vi "Read Logger.vi"(8 "error in (no error)":errorcluster, 11 "Log Message in":refnum<class "Log Message.lvclass">) -> (0 "error out":errorcluster, 2 "Logger":T1, 3 "Log Message out":refnum<class "Log Message.lvclass">)   [LabVIEW 2020, in "AIM MIL-STD-1553 Engine.lvlib" / "Implementation.lvlib" / "Word Logging.lvlib" / "Log Message.lvclass"]
uses:
  Log Message.lvclass
  Logger Data Reference.ctl
  Logger Interface/Logger Interface.lvclass
  Log Message.lvclass/Log Message.ctl
  Word Logging.lvlib
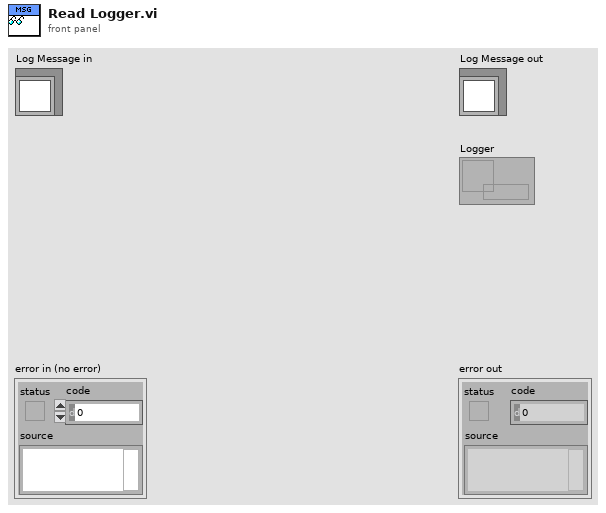
[diagram p1: front panel]
types:
  T1 = typedef "AIM MIL-STD-1553 Engine.lvlib/Implementation.lvlib/Word Logging.lvlib/Logger Data Reference.ctl" = refnum<data-value>
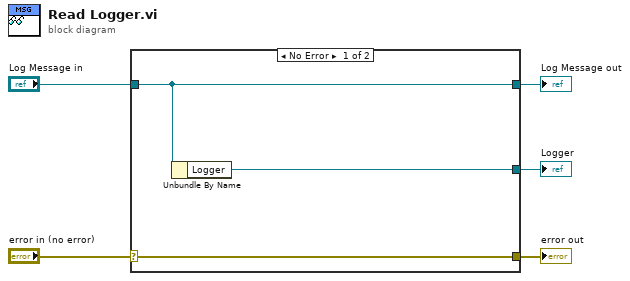
[diagram p0: block diagram]
diagram:
  n1 = case shown="No Error" "error in (no error)" {
    selector: "error in (no error)" -> [w8 w9]
    tunnel: [w8 w9] -> w4
    tunnel: [w7 w10] -> w2
    tunnel: "Log Message in" -> [w7 w10]
    tunnel: [w6 _] -> w1
    frame No Error {
      n2 = Unbundle By Name(w7) -> ("Logger"=w6:T1)
    }
    frame Error {
    }
  }
  "error out" <- w4
  "Log Message out" <- w2
  "Logger" <- w1
